vi "Shoot Switch.vi"(1 "Shoot Switch Long":bool, 2 "Shoot Switch Short":bool, 3 "error in (no error)":errorcluster) -> (10 "error out":errorcluster)   [LabVIEW 2017]
uses:
  Public/Documents/Cross The Road Electronics/Phoenix-LabVIEW/Motor Controller/Controls/CTRE_Phoenix_MotorControl_ControlMode.ctl
panel:
  # "NOTE: DOES NOT SEAT GEAR"
  # "Short: shoot -0.15\nLong: shoot -0.3"
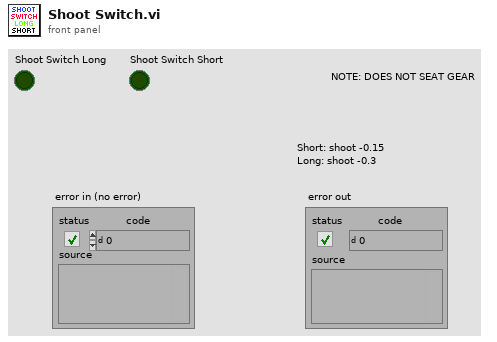
[diagram p1: front panel]
types:
  T1 = typedef "CTRE_Phoenix_MotorControl_ControlMode.ctl" = u16
  T2 = typedef "WPI_MotorControlDeviceRef.ctl" = cluster{"DeviceStatus":errorcluster, "Type":T3, "PWM":cluster{"PWM Channel":T4, "DeadBand":T5}, "CAN":cluster{"Device Number":u8, "SetOutput VI Ref":variant, "GetOutput VI Ref":variant, "Enable VI Ref":variant, "Disable VI Ref":variant, "Data":variant}, "Invert":bool, "DIO PWM":cluster{"PWM \"Enable\" Channel":T4, "DIOChannel":T6, "PWM Rate":dbl}}
  T3 = typedef "WPI_MotorControlType.ctl" = enum16{"PWM", "CAN", "DIO PWM"}
  T4 = typedef "FPGA_DIOPWMChannel.ctl" = enum8{"PWM 0", "PWM 1", "PWM 2", "PWM 3", "PWM 4", "PWM 5", "PWM 6", "PWM 7", "PWM 8", "PWM 9", "PWM MXP 0", "PWM MXP 1", "PWM MXP 2", "PWM MXP 3", "PWM MXP 4", "PWM MXP 5", "PWM MXP 6", "PWM MXP 7", "PWM MXP 8", "PWM MXP 9", "Invalid"}
  T5 = typedef "WPI_PWMDeadband.ctl" = cluster{"Name":string, "maxPositivePwm":i32, "minPositivePwm":i32, "centerPwm":i32, "maxNegativePwm":i32, "minNegativePwm":i32, "angularRange":u16}
  T6 = typedef "FPGA_DIOChannel.ctl" = enum8{"DIO 0", "DIO 1", "DIO 2", "DIO 3", "DIO 4", "DIO 5", "DIO 6", "DIO 7", "DIO 8", "DIO 9", "DIO MXP 0", "DIO MXP 1", "DIO MXP 2", "DIO MXP 3", "DIO MXP 4", "DIO MXP 5", "DIO MXP 6", "DIO MXP 7", "DIO MXP 8", "DIO MXP 9", "DIO MXP 10", "DIO MXP 11", "DIO MXP 12", "DIO MXP 13", "DIO MXP 14", "DIO MXP 15", "SPI Port CS1", "SPI Port CS2", "SPI Port CS3", "SPI Port MISO", "SPI Port MOSI", "Invalid"}
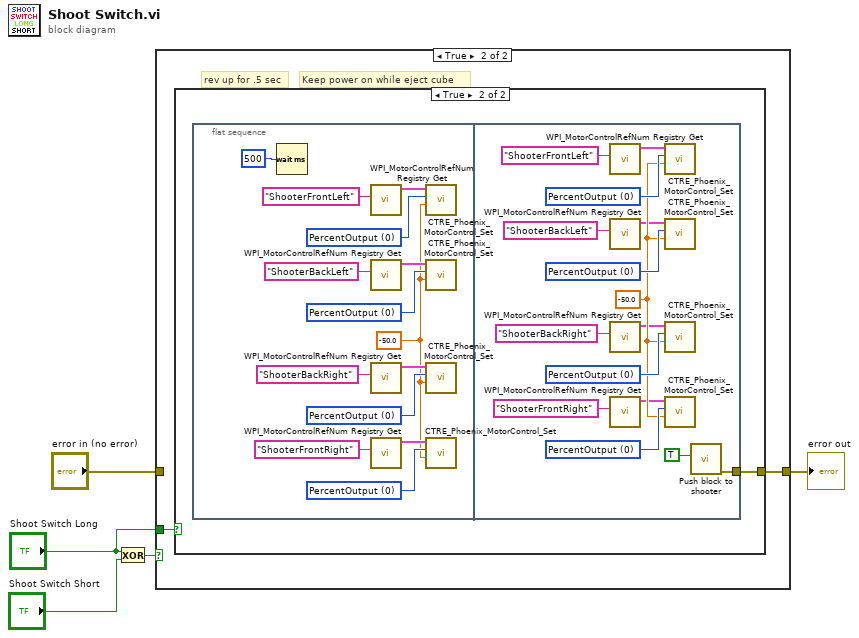
[diagram p0: block diagram]
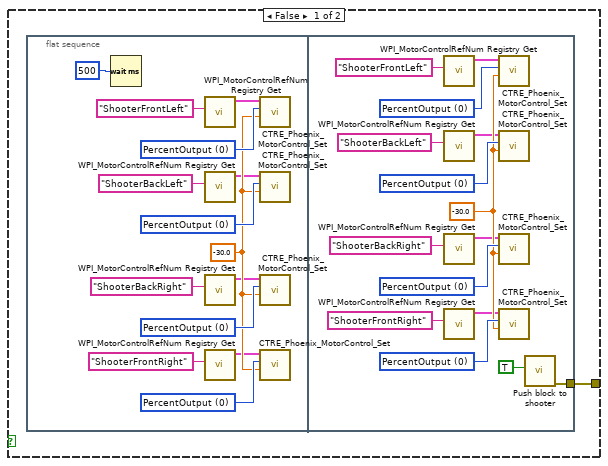
[diagram p3: hidden frame]
diagram:
  n1 = Exclusive Or(1:"Shoot Switch Short", 2:"Shoot Switch Long") -> (0:w5:bool)
  n2 = case shown="True" w5 {
    tunnel: "Shoot Switch Long" -> [_ w8]
    tunnel: "error in (no error)" -> [w6 _]
    tunnel: [w6 w7] -> w1
    frame False {
    }
    frame True {
      # "Keep power on while eject cube"
      # "rev up for .5 sec"
      n3 = case shown="True" w8 {
        tunnel: [w9 w39] -> w7
        frame False {
          n4 = flat-sequence {
            tunnel: [w37] -> w9
            frame #0 {
              w18 = -30.0
              w22 = T1 0 items=["PercentOutput"=0, "Position"=1, "Velocity"=2, "Current"=3, "Follower"=5, "MotionProfile"=6, "MotionMagic"=7, "MotionMagicArc"=8, "MotionProfileArc"=10, "Disabled"=15] ("Control Mode")
              w21 = T1 0 items=["PercentOutput"=0, "Position"=1, "Velocity"=2, "Current"=3, "Follower"=5, "MotionProfile"=6, "MotionMagic"=7, "MotionMagicArc"=8, "MotionProfileArc"=10, "Disabled"=15] ("Control Mode")
              w20 = T1 0 items=["PercentOutput"=0, "Position"=1, "Velocity"=2, "Current"=3, "Follower"=5, "MotionProfile"=6, "MotionMagic"=7, "MotionMagicArc"=8, "MotionProfileArc"=10, "Disabled"=15] ("Control Mode")
              w19 = T1 0 items=["PercentOutput"=0, "Position"=1, "Velocity"=2, "Current"=3, "Follower"=5, "MotionProfile"=6, "MotionMagic"=7, "MotionMagicArc"=8, "MotionProfileArc"=10, "Disabled"=15] ("Control Mode")
              n5 = Wait (ms)(milliseconds to wait=u32 500) -> ()  [unwired: 1 out]
              n6 = call <vilib>:"WPI_MotorControlRefNum Registry Get.vi"("refnum name"="ShooterFrontLeft") -> ("MotorControlDevRef"=w16:T2)  [unwired: 9 in, 1 out]
              n7 = call <vilib>:"WPI_MotorControlRefNum Registry Get.vi"("refnum name"="ShooterBackLeft") -> ("MotorControlDevRef"=w14:T2)  [unwired: 9 in, 1 out]
              n8 = call <vilib>:"WPI_MotorControlRefNum Registry Get.vi"("refnum name"="ShooterBackRight") -> ("MotorControlDevRef"=w13:T2)  [unwired: 9 in, 1 out]
              n9 = call <vilib>:"WPI_MotorControlRefNum Registry Get.vi"("refnum name"="ShooterFrontRight") -> ("MotorControlDevRef"=w11:T2)  [unwired: 9 in, 1 out]
              n10 = call "CTRE_Phoenix_MotorControl_Set.vi"("Output"=w18, "Control Mode"=w21, "PhoenixMotorControlDevRef"=w16) -> ()  [unwired: 7 in, 2 out]
              n11 = call "CTRE_Phoenix_MotorControl_Set.vi"("Output"=w18, "Control Mode"=w19, "PhoenixMotorControlDevRef"=w14) -> ()  [unwired: 7 in, 2 out]
              n12 = call "CTRE_Phoenix_MotorControl_Set.vi"("Output"=w18, "Control Mode"=w20, "PhoenixMotorControlDevRef"=w13) -> ()  [unwired: 7 in, 2 out]
              n13 = call "CTRE_Phoenix_MotorControl_Set.vi"("Output"=w18, "Control Mode"=w22, "PhoenixMotorControlDevRef"=w11) -> ()  [unwired: 7 in, 2 out]
            }
            frame #1 {
              w32 = -30.0
              w33 = T1 0 items=["PercentOutput"=0, "Position"=1, "Velocity"=2, "Current"=3, "Follower"=5, "MotionProfile"=6, "MotionMagic"=7, "MotionMagicArc"=8, "MotionProfileArc"=10, "Disabled"=15] ("Control Mode")
              w34 = T1 0 items=["PercentOutput"=0, "Position"=1, "Velocity"=2, "Current"=3, "Follower"=5, "MotionProfile"=6, "MotionMagic"=7, "MotionMagicArc"=8, "MotionProfileArc"=10, "Disabled"=15] ("Control Mode")
              w35 = T1 0 items=["PercentOutput"=0, "Position"=1, "Velocity"=2, "Current"=3, "Follower"=5, "MotionProfile"=6, "MotionMagic"=7, "MotionMagicArc"=8, "MotionProfileArc"=10, "Disabled"=15] ("Control Mode")
              w36 = T1 0 items=["PercentOutput"=0, "Position"=1, "Velocity"=2, "Current"=3, "Follower"=5, "MotionProfile"=6, "MotionMagic"=7, "MotionMagicArc"=8, "MotionProfileArc"=10, "Disabled"=15] ("Control Mode")
              n14 = call <vilib>:"WPI_MotorControlRefNum Registry Get.vi"("refnum name"="ShooterFrontLeft") -> ("MotorControlDevRef"=w31:T2)  [unwired: 9 in, 1 out]
              n15 = call <vilib>:"WPI_MotorControlRefNum Registry Get.vi"("refnum name"="ShooterBackLeft") -> ("MotorControlDevRef"=w30:T2)  [unwired: 9 in, 1 out]
              n16 = call <vilib>:"WPI_MotorControlRefNum Registry Get.vi"("refnum name"="ShooterBackRight") -> ("MotorControlDevRef"=w29:T2)  [unwired: 9 in, 1 out]
              n17 = call <vilib>:"WPI_MotorControlRefNum Registry Get.vi"("refnum name"="ShooterFrontRight") -> ("MotorControlDevRef"=w28:T2)  [unwired: 9 in, 1 out]
              n18 = call "CTRE_Phoenix_MotorControl_Set.vi"("Output"=w32, "Control Mode"=w34, "PhoenixMotorControlDevRef"=w31) -> ()  [unwired: 7 in, 2 out]
              n19 = call "CTRE_Phoenix_MotorControl_Set.vi"("Output"=w32, "Control Mode"=w36, "PhoenixMotorControlDevRef"=w30) -> ()  [unwired: 7 in, 2 out]
              n20 = call "CTRE_Phoenix_MotorControl_Set.vi"("Output"=w32, "Control Mode"=w35, "PhoenixMotorControlDevRef"=w29) -> ()  [unwired: 7 in, 2 out]
              n21 = call "CTRE_Phoenix_MotorControl_Set.vi"("Output"=w32, "Control Mode"=w33, "PhoenixMotorControlDevRef"=w28) -> ()  [unwired: 7 in, 2 out]
              n22 = call "Push block to shooter.vi"("Shoot?"=TRUE) -> ("error out"=w37:errorcluster)  [unwired: 10 in]
            }
          }
        }
        frame True {
          n23 = flat-sequence {
            tunnel: [w67] -> w39
            frame #0 {
              w40 = -50.0
              w48 = T1 0 items=["PercentOutput"=0, "Position"=1, "Velocity"=2, "Current"=3, "Follower"=5, "MotionProfile"=6, "MotionMagic"=7, "MotionMagicArc"=8, "MotionProfileArc"=10, "Disabled"=15] ("Control Mode")
              w47 = T1 0 items=["PercentOutput"=0, "Position"=1, "Velocity"=2, "Current"=3, "Follower"=5, "MotionProfile"=6, "MotionMagic"=7, "MotionMagicArc"=8, "MotionProfileArc"=10, "Disabled"=15] ("Control Mode")
              w46 = T1 0 items=["PercentOutput"=0, "Position"=1, "Velocity"=2, "Current"=3, "Follower"=5, "MotionProfile"=6, "MotionMagic"=7, "MotionMagicArc"=8, "MotionProfileArc"=10, "Disabled"=15] ("Control Mode")
              w45 = T1 0 items=["PercentOutput"=0, "Position"=1, "Velocity"=2, "Current"=3, "Follower"=5, "MotionProfile"=6, "MotionMagic"=7, "MotionMagicArc"=8, "MotionProfileArc"=10, "Disabled"=15] ("Control Mode")
              n24 = Wait (ms)(milliseconds to wait=u32 500) -> ()  [unwired: 1 out]
              n25 = call <vilib>:"WPI_MotorControlRefNum Registry Get.vi"("refnum name"="ShooterFrontLeft") -> ("MotorControlDevRef"=w42:T2)  [unwired: 9 in, 1 out]
              n26 = call <vilib>:"WPI_MotorControlRefNum Registry Get.vi"("refnum name"="ShooterBackLeft") -> ("MotorControlDevRef"=w44:T2)  [unwired: 9 in, 1 out]
              n27 = call <vilib>:"WPI_MotorControlRefNum Registry Get.vi"("refnum name"="ShooterBackRight") -> ("MotorControlDevRef"=w43:T2)  [unwired: 9 in, 1 out]
              n28 = call <vilib>:"WPI_MotorControlRefNum Registry Get.vi"("refnum name"="ShooterFrontRight") -> ("MotorControlDevRef"=w41:T2)  [unwired: 9 in, 1 out]
              n29 = call "CTRE_Phoenix_MotorControl_Set.vi"("Output"=w40, "Control Mode"=w47, "PhoenixMotorControlDevRef"=w42) -> ()  [unwired: 7 in, 2 out]
              n30 = call "CTRE_Phoenix_MotorControl_Set.vi"("Output"=w40, "Control Mode"=w45, "PhoenixMotorControlDevRef"=w44) -> ()  [unwired: 7 in, 2 out]
              n31 = call "CTRE_Phoenix_MotorControl_Set.vi"("Output"=w40, "Control Mode"=w46, "PhoenixMotorControlDevRef"=w43) -> ()  [unwired: 7 in, 2 out]
              n32 = call "CTRE_Phoenix_MotorControl_Set.vi"("Output"=w40, "Control Mode"=w48, "PhoenixMotorControlDevRef"=w41) -> ()  [unwired: 7 in, 2 out]
            }
            frame #1 {
              w62 = -50.0
              w66 = T1 0 items=["PercentOutput"=0, "Position"=1, "Velocity"=2, "Current"=3, "Follower"=5, "MotionProfile"=6, "MotionMagic"=7, "MotionMagicArc"=8, "MotionProfileArc"=10, "Disabled"=15] ("Control Mode")
              w65 = T1 0 items=["PercentOutput"=0, "Position"=1, "Velocity"=2, "Current"=3, "Follower"=5, "MotionProfile"=6, "MotionMagic"=7, "MotionMagicArc"=8, "MotionProfileArc"=10, "Disabled"=15] ("Control Mode")
              w64 = T1 0 items=["PercentOutput"=0, "Position"=1, "Velocity"=2, "Current"=3, "Follower"=5, "MotionProfile"=6, "MotionMagic"=7, "MotionMagicArc"=8, "MotionProfileArc"=10, "Disabled"=15] ("Control Mode")
              w63 = T1 0 items=["PercentOutput"=0, "Position"=1, "Velocity"=2, "Current"=3, "Follower"=5, "MotionProfile"=6, "MotionMagic"=7, "MotionMagicArc"=8, "MotionProfileArc"=10, "Disabled"=15] ("Control Mode")
              n33 = call <vilib>:"WPI_MotorControlRefNum Registry Get.vi"("refnum name"="ShooterFrontLeft") -> ("MotorControlDevRef"=w56:T2)  [unwired: 9 in, 1 out]
              n34 = call <vilib>:"WPI_MotorControlRefNum Registry Get.vi"("refnum name"="ShooterBackLeft") -> ("MotorControlDevRef"=w54:T2)  [unwired: 9 in, 1 out]
              n35 = call <vilib>:"WPI_MotorControlRefNum Registry Get.vi"("refnum name"="ShooterBackRight") -> ("MotorControlDevRef"=w55:T2)  [unwired: 9 in, 1 out]
              n36 = call <vilib>:"WPI_MotorControlRefNum Registry Get.vi"("refnum name"="ShooterFrontRight") -> ("MotorControlDevRef"=w57:T2)  [unwired: 9 in, 1 out]
              n37 = call "CTRE_Phoenix_MotorControl_Set.vi"("Output"=w62, "Control Mode"=w65, "PhoenixMotorControlDevRef"=w56) -> ()  [unwired: 7 in, 2 out]
              n38 = call "CTRE_Phoenix_MotorControl_Set.vi"("Output"=w62, "Control Mode"=w63, "PhoenixMotorControlDevRef"=w54) -> ()  [unwired: 7 in, 2 out]
              n39 = call "CTRE_Phoenix_MotorControl_Set.vi"("Output"=w62, "Control Mode"=w64, "PhoenixMotorControlDevRef"=w55) -> ()  [unwired: 7 in, 2 out]
              n40 = call "CTRE_Phoenix_MotorControl_Set.vi"("Output"=w62, "Control Mode"=w66, "PhoenixMotorControlDevRef"=w57) -> ()  [unwired: 7 in, 2 out]
              n41 = call "Push block to shooter.vi"("Shoot?"=TRUE) -> ("error out"=w67:errorcluster)  [unwired: 10 in]
            }
          }
        }
      }
    }
  }
  "error out" <- w1
